vi "PID Auto Drive.vi"(8 "Targets":T1, 9 "Motor Values":T5, 10 "Tolerances":T4, 11 "PID Gains":T3={"Gyro PID Gains"={"proportional gain (Kc)"=1.0, "integral time (Ti, min)"=0.01, "derivative time (Td, min)"=0.0}, "Distance PID Gains"={"proportional gain (Kc)"=1.0, "integral time (Ti, min)"=0.01, "derivative time (Td, min)"=0.0}, "Strafe PID Gains"={"proportional gain (Kc)"=1.0, "integral time (Ti, min)"=0.01, "derivative time (Td, min)"=0.0}} {"Strafe PID Gains"."derivative time (Td, min)" format="%.3f"; "Strafe PID Gains"."integral time (Ti, min)" format="%.3f"; "Strafe PID Gains"."proportional gain (Kc)" format="%.3f"; "Distance PID Gains"."derivative time (Td, min)" format="%.3f"; "Distance PID Gains"."integral time (Ti, min)" format="%.3f"; "Distance PID Gains"."proportional gain (Kc)" format="%.3f"; "Gyro PID Gains"."derivative time (Td, min)" format="%.3f"; "Gyro PID Gains"."integral time (Ti, min)" format="%.3f"; "Gyro PID Gains"."proportional gain (Kc)" format="%.3f"}) -> (0 "Center Piston Down?":bool, 1 "Z Out":dbl, 2 "X Out":dbl, 3 "Y Out":dbl, 4 "Finished?":bool)   [LabVIEW 2016]
uses:
  Common Code/PID Gains.ctl
  Common Code/Utilities/Change Detect Double.vi
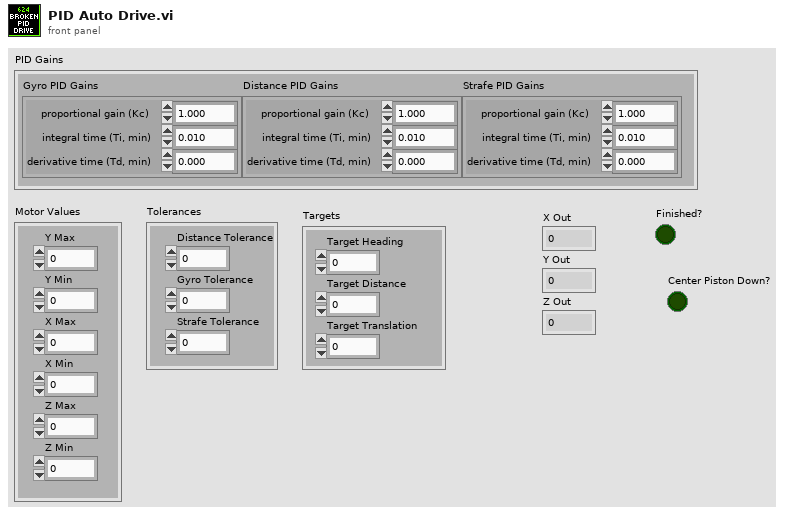
[diagram p1: front panel]
types:
  T1 = cluster{"Target Heading":dbl, "Target Distance":dbl, "Target Translation":dbl}
  T2 = typedef "PID Gains.ctl" = cluster{"proportional gain (Kc)":dbl, "integral time (Ti, min)":dbl, "derivative time (Td, min)":dbl}
  T3 = cluster{"Gyro PID Gains":T2, "Distance PID Gains":T2, "Strafe PID Gains":T2}
  T4 = cluster{"Distance Tolerance":dbl, "Strafe Tolerance":dbl, "Gyro Tolerance":dbl}
  T5 = cluster{"Y Max":dbl, "X Max":dbl, "Z Max":dbl, "Y Min":dbl, "X Min":dbl, "Z Min":dbl}
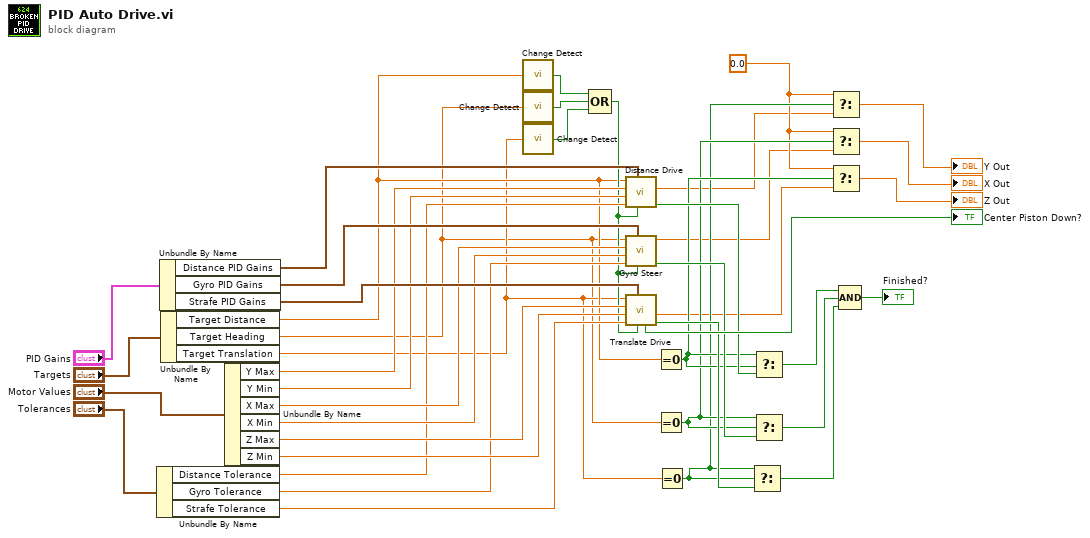
[diagram p0: block diagram]
diagram:
  w7 = 0.0 ("t")
  n1 = Unbundle By Name("Tolerances") -> ("Distance Tolerance"=w27:dbl, "Gyro Tolerance"=w26:dbl, "Strafe Tolerance"=w28:dbl)
  n2 = Unbundle By Name("PID Gains") -> ("Distance PID Gains"=w37:T2, "Gyro PID Gains"=w36:T2, "Strafe PID Gains"=w35:T2)
  n3 = Unbundle By Name("Targets") -> ("Target Distance"=w19:dbl, "Target Heading"=w11:dbl, "Target Translation"=w18:dbl)
  n4 = Unbundle By Name("Motor Values") -> ("Y Max"=w34:dbl, "Y Min"=w33:dbl, "X Max"=w32:dbl, "X Min"=w31:dbl, "Z Max"=w30:dbl, "Z Min"=w29:dbl)
  n5 = call-poly "Change Detect.vi"("In"=w19) -> ("Changed?"=w25:bool)
  n6 = call-poly "Change Detect.vi"("In"=w11) -> ("Changed?"=w24:bool)
  n7 = call-poly "Change Detect.vi"("In"=w18) -> ("Changed?"=w23:bool)
  n8 = Compound Arithmetic op=OR(w25, w24, w23) -> (w22:bool)
  n9 = call "Distance Drive.vi"("Reinit?"=w22, "PID gains"=w37, "Distance Tolerance"=w27, "Y Min Output"=w33, "Y Max Output"=w34, "Distance Target"=w19) -> ("Finished?"=w16:bool, "Y Output"=w6:dbl)  [unwired: 4 in]
  n10 = call "Gyro Steer.vi"("Reinit?"=w22, "PID gains"=w36, "Gyro Tolerance"=w26, "X Min Output"=w31, "X Max Output"=w32, "Target Heading"=w11) -> ("Finished?"=w13:bool, "X out"=w5:dbl)  [unwired: 4 in]
  n11 = call "Translate Drive.vi"("Reinit?"=w22, "Translation PID Gains"=w35, "Translation Tolerance"=w28, "Z Min Output"=w29, "Z Max Output"=w30, "Target Translation"=w18) -> ("Finished?"=w15:bool, "Z Out"=w4:dbl, "Center Piston Down?"=→"Center Piston Down?":bool)  [unwired: 3 in]
  n12 = Equal To 0?(x=w19) -> (x = 0?=w10:bool)
  n13 = Equal To 0?(x=w11) -> (x = 0?=w9:bool)
  n14 = Equal To 0?(x=w18) -> (x = 0?=w8:bool)
  n15 = Select(t=w8, s=w8, f=w15) -> (s? t:f=w14:bool)
  n16 = Select(t=w10, s=w10, f=w16) -> (s? t:f=w17:bool)
  n17 = Select(t=w9, s=w9, f=w13) -> (s? t:f=w12:bool)
  n18 = Select(t=w7, s=w8, f=w6) -> (s? t:f=→"Y Out":dbl)
  n19 = Select(t=w7, s=w9, f=w5) -> (s? t:f=→"X Out":dbl)
  n20 = Select(t=w7, s=w10, f=w4) -> (s? t:f=→"Z Out":dbl)
  n21 = Compound Arithmetic op=AND(w17, w12, w14) -> (→"Finished?":bool)
